vi "Create Optical Flow Source Images(SubVI).vi"(8 "error in (no error)":errorcluster) -> (0 "error out":errorcluster, 1 "Optical Flow Velocity X":T1, 2 "Optical Flow Previous Image":T1, 3 "Optical Flow Velocity Y":T1, 4 "Optical Flow Current Image":T1, 5 "Raw input":T1)   [LabVIEW 2014]
uses:
  <vilib>/vision/Image Controls.llb/IMAQ Image.ctl
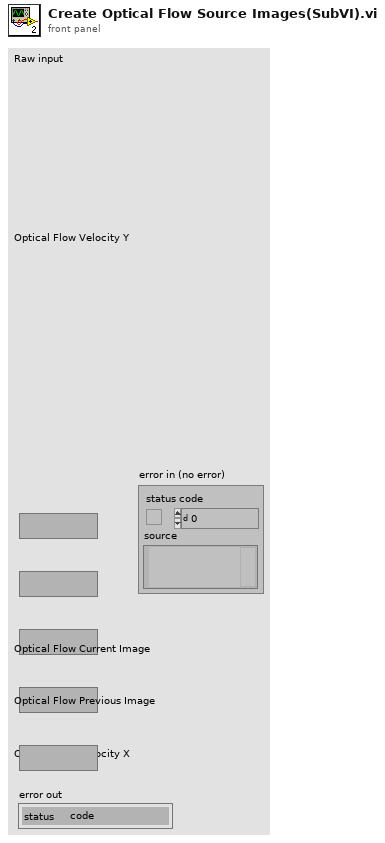
[diagram p1: front panel]
types:
  T1 = typedef "IMAQ Image.ctl" = refnum<image>
  T2 = typedef "Image Type" = u32
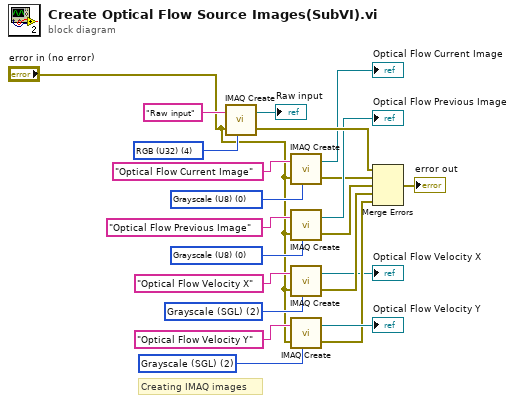
[diagram p0: block diagram]
diagram:
  w20 = T2 4 items=["Grayscale (U8)", "Grayscale (I16)", "Grayscale (SGL)", "Complex (CSG)", "RGB (U32)", "HSL (U32)", "RGB (U64)", "Grayscale (U16)"] ("Image Type")
  w10 = T2 2 items=["Grayscale (U8)", "Grayscale (I16)", "Grayscale (SGL)", "Complex (CSG)", "RGB (U32)", "HSL (U32)", "RGB (U64)", "Grayscale (U16)"] ("Image Type")
  w9 = T2 0 items=["Grayscale (U8)", "Grayscale (I16)", "Grayscale (SGL)", "Complex (CSG)", "RGB (U32)", "HSL (U32)", "RGB (U64)", "Grayscale (U16)"] ("Image Type")
  w8 = T2 0 items=["Grayscale (U8)", "Grayscale (I16)", "Grayscale (SGL)", "Complex (CSG)", "RGB (U32)", "HSL (U32)", "RGB (U64)", "Grayscale (U16)"] ("Image Type")
  w7 = T2 2 items=["Grayscale (U8)", "Grayscale (I16)", "Grayscale (SGL)", "Complex (CSG)", "RGB (U32)", "HSL (U32)", "RGB (U64)", "Grayscale (U16)"] ("Image Type")
  # "Creating IMAQ images"
  n1 = call "IMAQ Create"("Image Name"="Raw input", "Image Type"=w20, "error in (no error)"="error in (no error)") -> ("New Image"=→"Raw input":T1, "error out"=w22:errorcluster)  [unwired: 1 in, 1 out]
  n2 = call "IMAQ Create"("Image Name"="Optical Flow Current Image", "Image Type"=w8, "error in (no error)"="error in (no error)") -> ("New Image"=→"Optical Flow Current Image":T1, "error out"=w11:errorcluster)  [unwired: 1 in, 1 out]
  n3 = call "IMAQ Create"("Image Name"="Optical Flow Previous Image", "Image Type"=w9, "error in (no error)"="error in (no error)") -> ("New Image"=→"Optical Flow Previous Image":T1, "error out"=w12:errorcluster)  [unwired: 1 in, 1 out]
  n4 = call "IMAQ Create"("Image Name"="Optical Flow Velocity X", "Image Type"=w7, "error in (no error)"="error in (no error)") -> ("New Image"=→"Optical Flow Velocity X":T1, "error out"=w13:errorcluster)  [unwired: 1 in, 1 out]
  n5 = call "IMAQ Create"("Image Name"="Optical Flow Velocity Y", "Image Type"=w10, "error in (no error)"="error in (no error)") -> ("New Image"=→"Optical Flow Velocity Y":T1, "error out"=w14:errorcluster)  [unwired: 1 in, 1 out]
  n6 = Merge Errors(w22, w11, w12, w13, w14) -> (→"error out":errorcluster)
